vi "Create DefaultReport.vi"(6 "Verbose":bool, 8 "error in (no error)":errorcluster, 10 "Report Path":path, 11 "Test Report.Default in":refnum<class "Test Report.Default.lvclass">) -> (0 "error out":errorcluster, 3 "Test Report.Default out":refnum<class "Test Report.Default.lvclass">)   [LabVIEW 2013, in "Caraya.lvlib" / "Test Report.Default.lvclass"]
uses:
  Test Report.Default.lvclass
  Test Report/Test Report.lvclass/Test Report.ctl
  Test Report/Test Report.lvclass
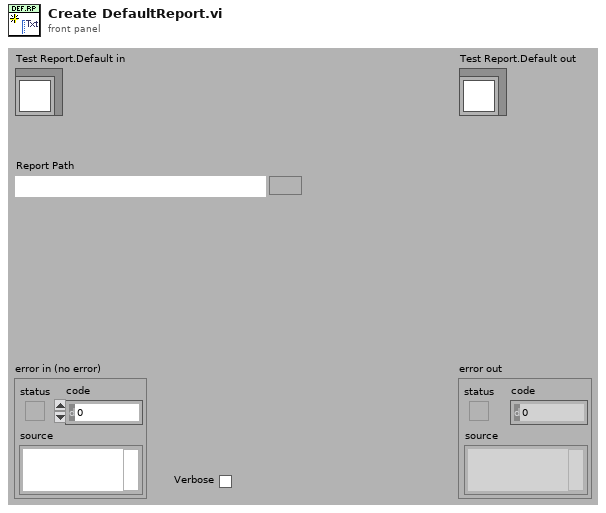
[diagram p1: front panel]
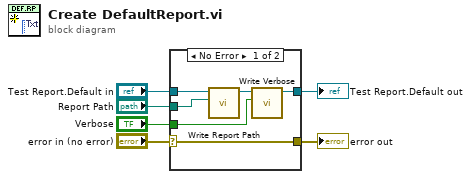
[diagram p0: block diagram]
diagram:
  n1 = case shown="No Error" "error in (no error)" {
    selector: "error in (no error)" -> [w10 w13]
    tunnel: "Test Report.Default in" -> [w12 w14]
    tunnel: [w8 w14] -> w5
    tunnel: "Report Path" -> [w11 _]
    tunnel: [w10 w13] -> w2
    tunnel: "Verbose" -> [w7 _]
    frame No Error {
      n2 = call "Write Report Path.vi"("Report Path"=w11, "Test Report.Default in"=w12) -> ("Test Report.Default out"=w9:refnum<class "Test Report.Default.lvclass">)  [unwired: 9 in]
      n3 = call "Write Verbose.vi"("Verbose"=w7, "Test Report in"=w9) -> ("Test Report out"=w8:refnum<class "Test Report.Default.lvclass">)  [unwired: 8 in, 1 out]
    }
    frame Error {
    }
  }
  "error out" <- w2
  "Test Report.Default out" <- w5
